vi "config-NTR.vi"() -> ()   [LabVIEW 2024]
uses:
  controls/UiNutritionPanel.ctl
  controls/UiScheduleTimestamp.ctl
  <vilib>/Utility/miscctls.llb/LVPointTypeDef.ctl
  controls/typePathSelector.ctl
  globals/globals-engine.vi
panel:
  in  "Index":u8=1 min=1 max=16 step=1
  in  "DataChanged?":bool=TRUE
  in  "Reload":bool
  in  "Save":bool
  in  "conf in":T1[](array[typedef]) {"ORP Dosing"."MIX Limit" format="%d [s]"; "ORP Dosing"."MIX Dose" format="%d [s]"; "PH Dosing"."ACID Limit" format="%d [s]"; "PH Dosing"."BASE Limit" format="%d [s]"; "PH Dosing"."ACID Dose" format="%d [s]"; "PH Dosing"."BASE Dose" format="%d [s]"; "EC Dosing"."BETA2 Limit" format="%d [s]"; "EC Dosing"."ALFA2 Limit" format="%d [s]"; "EC Dosing"."ALFA2 Dose" format="%d [s]"; "EC Dosing"."BETA2 Dose" format="%d [s]"; "EC Dosing"."BETA1 Limit" format="%d [s]"; "EC Dosing"."ALFA1 Limit" format="%d [s]"; "EC Dosing"."ALFA1 Dose" format="%d [s]"; "EC Dosing"."BETA1 Dose" format="%d [s]"; "Main"."DailyActivityHours"."Begin Time" format="ON:    %<%H:%M>T"; "Main"."DailyActivityHours"."End Time" format="OFF:    %<%H:%M>T"; "Main"."WashTimes"."Out" format="Wash out: %d [sec]"; "Main"."WashTimes"."In" format="Wash in: %d [sec]"; "Water Dosing"."Water Limit" format="%d [s]"; "Water Dosing"."Water Dose" format="%d [s]"}
  # "Water"
  # "EC"
  # "PH"
  # "ORP"
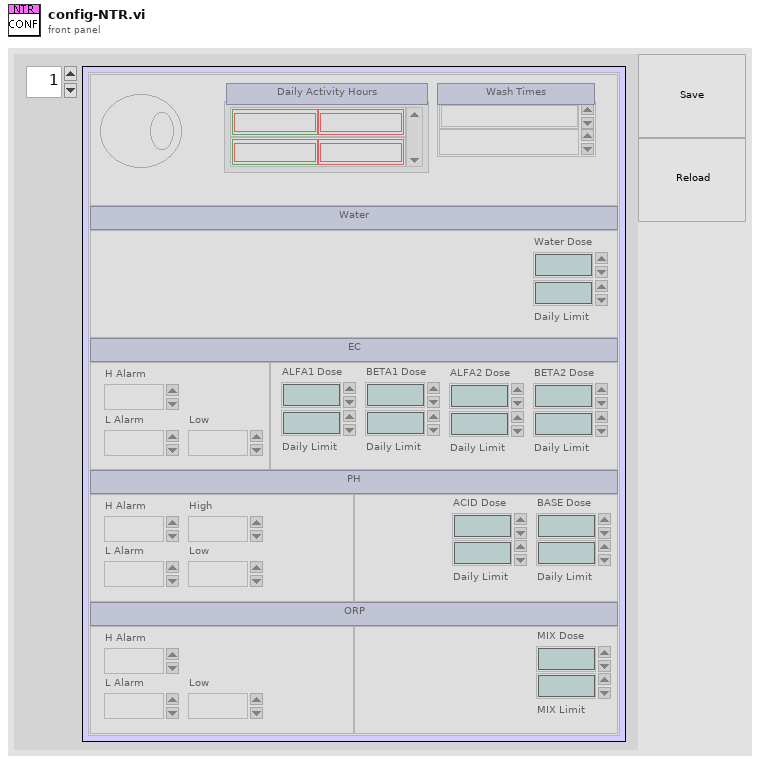
[diagram p1: front panel]
types:
  T1 = typedef "UiNutritionPanel.ctl" = cluster{"Main":cluster{"Enable":bool, "WashTimes":cluster{"In":dbl, "Out":dbl}, "DailyActivityHours":cluster{"Begin Time":T2, "End Time":T2}[]}, "Water Dosing":cluster{"Water Dose":dbl, "Water Limit":dbl}, "EC Ranges":cluster{"H Alarm":dbl, "L Alarm":dbl, "Low":dbl}, "EC Dosing":cluster{"ALFA1 Dose":dbl, "ALFA1 Limit":dbl, "BETA1 Dose":dbl, "BETA1 Limit":dbl, "ALFA2 Dose":dbl, "ALFA2 Limit":dbl, "BETA2 Dose":dbl, "BETA2 Limit":dbl}, "PH Ranges":cluster{"H Alarm":dbl, "L Alarm":dbl, "High":dbl, "Low":dbl}, "PH Dosing":cluster{"ACID Dose":dbl, "ACID Limit":dbl, "BASE Dose":dbl, "BASE Limit":dbl}, "ORP Ranges":cluster{"H Alarm":dbl, "L Alarm":dbl, "Low":dbl}, "ORP Dosing":cluster{"MIX Dose":dbl, "MIX Limit":dbl}}
  T2 = typedef "UiScheduleTimestamp.ctl" = timestamp
  T3 = typedef "typePathSelector.ctl" = enum16{"DIR_PROCS", "DIR_CONFIG", "DIR_TEMPLATE", "DIR_IO_FILE", "DIR_RECORD", "DIR_LOG", "DIR_RUNTIME", "DIR_PRESET", "DIR_INI"}
  T4 = typedef "LVPointTypeDef.ctl" = cluster{"Horizontal":i16, "Vertical":i16}
  T5 = enum32{"Invalid", "Standard", "Closed", "Hidden", "Minimized", "Maximized"}
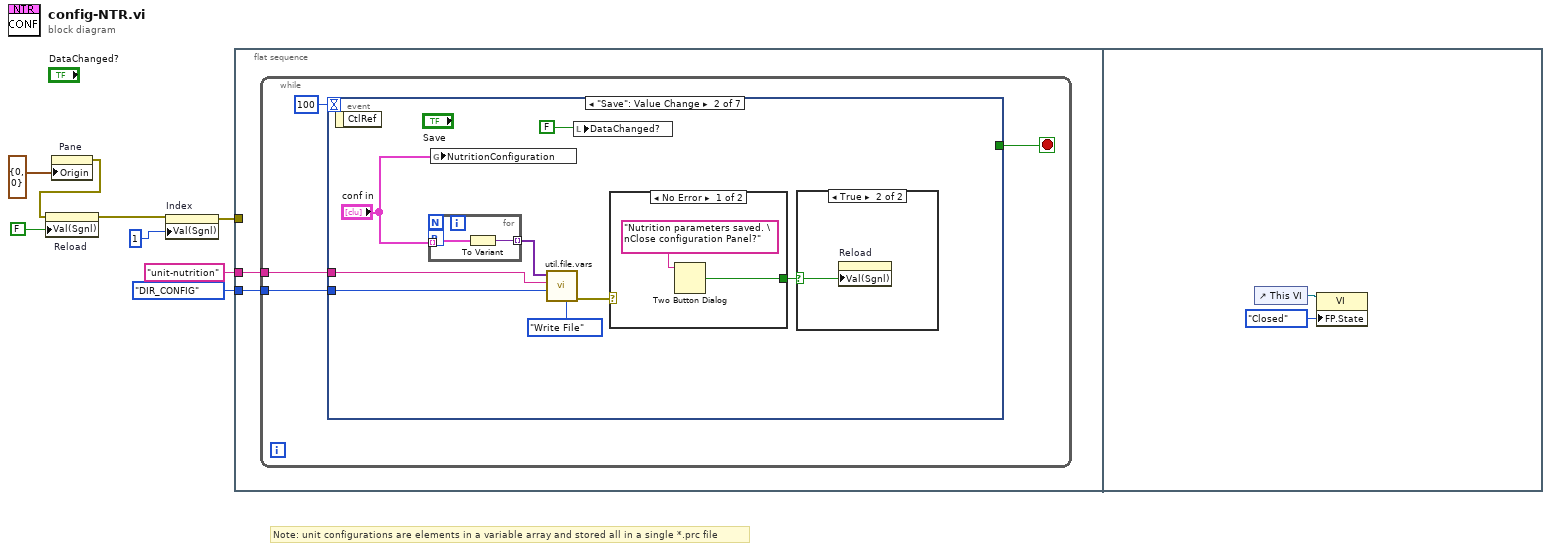
[diagram p0: block diagram]
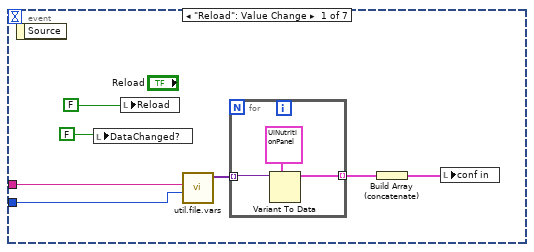
[diagram p2: hidden frame]
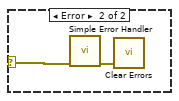
[diagram p4: hidden frame]
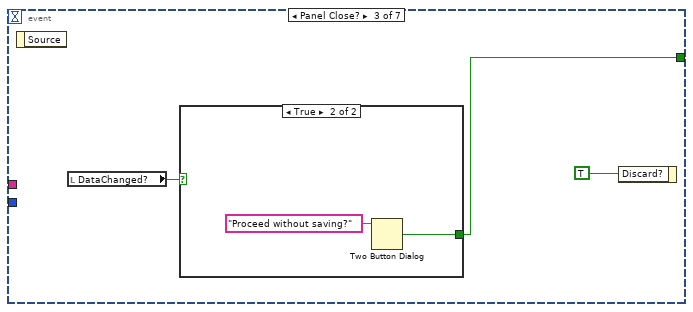
[diagram p5: hidden frame]
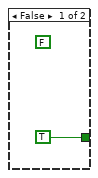
[diagram p6: hidden frame]
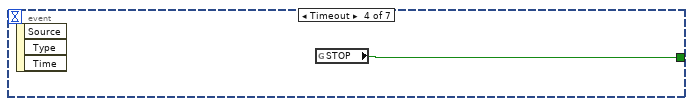
[diagram p7: hidden frame]
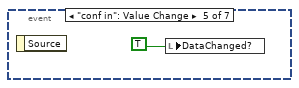
[diagram p8: hidden frame]
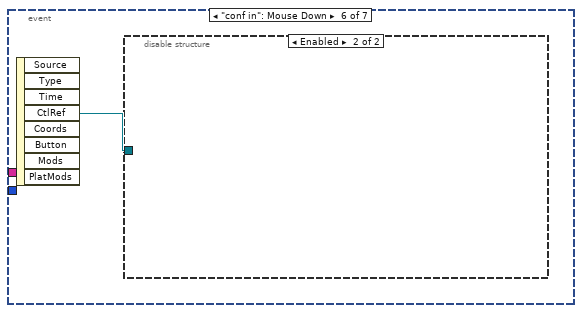
[diagram p9: hidden frame]
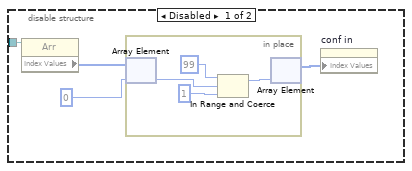
[diagram p10: hidden frame]
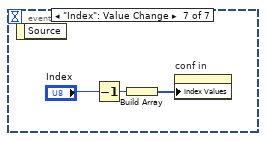
[diagram p11: hidden frame]
diagram:
  # "Note: unit configurations are elements in a variable array and stored all in a single *.prc file"
  n1 = property on="Pane" class="Pane"("Origin"=T4 {"Horizontal"=0, "Vertical"=0}) -> (error out=w1:errorcluster)  [unwired: 2 in, 1 out]
  n2 = property on="Reload" class="Bool (strict)"(error in=w1, "Val(Sgnl)"=FALSE ("Value (Signaling)")) -> (error out=w2:errorcluster)  [unwired: 1 in, 1 out]
  n3 = property on="Index" class="DigNum (strict)"(error in=w2, "Val(Sgnl)"=u8 1 ("Numeric")) -> (error out=w3:errorcluster)  [unwired: 1 in, 1 out]
  n4 = flat-sequence {
    tunnel: typePathSelector."DIR_CONFIG" ("location (PROCEDURE_DIR)") -> [w10]
    tunnel: "unit-nutrition" ("Filename.*  (opens dialog if empty and allow)") -> [w9]
    tunnel: w3 -> [_]
    frame #0 {
      n5 = while {
        tunnel: w10 -> [w14]
        tunnel: w9 -> [w13]
        stop <- w12 stop-if-true
        n6 = event shown="[1] \"Save\": Value Change" {
          selector: _ -> [_ _ _ _ _ _ _]
          dyn-events: _ -> [_ _ _ _ _ _ _]
          timeout: 100 -> [_ _ _ _ _ _ _]
          tunnel: w14 -> [w21 w31 _ _ _ _ _]
          tunnel: w13 -> [w20 w30 _ _ _ _ _]
          tunnel: [_ _ w41 w46 _ _ _] -> w12
          event "Reload": Value Change {
            n7 = event-data() -> ()  [unwired: 1 in, 1 out]
            n8 = local write "DataChanged?"(FALSE ("Value (Signaling)")) -> ()
            n9 = local write "Reload"(FALSE ("Reload")) -> ()
            n10 = call "util.file.vars.vi"("Directory (DIR_PROC)"=w21, "Proc Name(open dialog if empty)"=w20) -> ("Vars[] out"=w19:variant[])  [unwired: 5 in, 4 out]
            n11 = for {
              tunnel: w19 -> [w24] mode=indexing
              tunnel: [w23] -> w18 mode=indexing
              n12 = Variant To Data(type=T1 {"Main"={"Enable"=FALSE, "WashTimes"={"In"=0.0, "Out"=0.0}, "DailyActivityHours"=[]}, "Water Dosing"={"Water Dose"=0.0, "Water Limit"=0.0}, "EC Ranges"={"H Alarm"=0.0, "L Alarm"=0.0, "Low"=0.0}, "EC Dosing"={"ALFA1 Dose"=0.0, "ALFA1 Limit"=0.0, "BETA1 Dose"=0.0, "BETA1 Limit"=0.0, "ALFA2 Dose"=0.0, "ALFA2 Limit"=0.0, "BETA2 Dose"=0.0, "BETA2 Limit"=0.0}, "PH Ranges"={"H Alarm"=0.0, "L Alarm"=0.0, "High"=0.0, "Low"=0.0}, "PH Dosing"={"ACID Dose"=0.0, "ACID Limit"=0.0, "BASE Dose"=0.0, "BASE Limit"=0.0}, "ORP Ranges"={"H Alarm"=0.0, "L Alarm"=0.0, "Low"=0.0}, "ORP Dosing"={"MIX Dose"=0.0, "MIX Limit"=0.0}} ("Cluster"), Variant=w24) -> (data=w23:T1)  [unwired: 1 in, 1 out]
            }
            n13 = Build Array (concatenate)(w18) -> (w15:T1[])
            n14 = local write "conf in"(w15) -> ()
          }
          event "Save": Value Change {
            n15 = event-data() -> ()  [unwired: 1 in, 1 out]
            n16 = for {
              tunnel: "conf in" -> [w39] mode=indexing
              tunnel: [w38] -> w32 mode=indexing
              workers-P: _ -> [_]
              n17 = To Variant(anything=w39) -> (Variant=w38:variant)
            }
            n18 = global write "globals-engine.vi" "NutritionConfiguration"("conf in") -> ()
            n19 = call "util.file.vars.vi"("Operation(Read)"=enum16{"Read File", "Write File"}."Write File", "Directory (DIR_PROC)"=w31, "Proc Name(open dialog if empty)"=w30, "Vars[] in"=w32) -> ("error out"=w28:errorcluster)  [unwired: 3 in, 4 out]
            n20 = local write "DataChanged?"(FALSE ("Value (Signaling)")) -> ()
            n21 = case shown="No Error" w28 {
              selector: w28 -> [_ w37]
              tunnel: [w34 _] -> w27
              frame No Error {
                n22 = Two Button Dialog(message="Nutrition parameters saved. \nClose configuration Panel?") -> (T button?=w34:bool)  [unwired: 2 in]
              }
              frame Error {
                n23 = call <vilib>:"Simple Error Handler.vi"("error in (no error)"=w37) -> ("error out"=w36:errorcluster)  [unwired: 4 in, 4 out]
                n24 = call <vilib>:"Clear Errors.vi"("error in (no error)"=w36) -> ()  [unwired: 5 in, 2 out]
              }
            }
            n25 = case shown="True" w27 {
              selector: w27 -> [_ w33]
              frame False {
              }
              frame True {
                n26 = property on="Reload" class="Bool (strict)"("Val(Sgnl)"=w33) -> ()  [unwired: 2 in, 2 out]
              }
            }
          }
          event Panel Close? {
            n27 = event-data() -> ()  [unwired: 1 in, 1 out]
            n28 = local read "DataChanged?"() -> (w42:bool)
            n29 = case shown="True" w42 {
              tunnel: [TRUE ("T button?") w44] -> w41
              frame False {
                (unwired) FALSE ("T button?")
              }
              frame True {
                n30 = Two Button Dialog(message="Proceed without saving?") -> (T button?=w44:bool)  [unwired: 2 in]
              }
            }
            n31 = event-data("Discard?"=TRUE) -> ()  [unwired: 1 in, 1 out]
          }
          event Timeout {
            n32 = event-data() -> ()  [unwired: 1 in, 3 out]
            n33 = global read "globals-engine.vi" "STOP"() -> (w46:bool)
          }
          event "conf in": Value Change {
            n34 = event-data() -> ()  [unwired: 1 in, 1 out]
            n35 = local write "DataChanged?"(TRUE ("Value (Signaling)")) -> ()
          }
          event "conf in": Mouse Down {
            n36 = event-data() -> ("CtlRef"=w48:refnum<vi>)  [unwired: 1 in, 7 out]
            n37 = disable-structure shown="Enabled" {
              disable-tunnel: w48 -> [w50 _]
              frame Disabled {
                n38 = property class="Arr"(reference=w50) -> ("Index Values"=w49:u32[])  [unwired: 1 in, 2 out]
                n39 = in-place {
                  n40 = in-place-array #1(w49, 0) -> (w56:u32)
                  n41 = In Range and Coerce(upper limit=99, x=w56, lower limit=u32 1) -> (coerced(x)=w54:u32)  [unwired: 1 out]
                  n42 = in-place-array #1(w54) -> (w51:u32[])  [unwired: 1 out]
                }
                n43 = property on="conf in" class="Arr"("Index Values"=w51) -> ()  [unwired: 2 in, 2 out]
              }
              frame Enabled {
              }
            }
          }
          event "Index": Value Change {
            n44 = event-data() -> ()  [unwired: 1 in, 1 out]
            n45 = Decrement(x="Index") -> (x-1=w57:u8)
            n46 = Build Array(w57) -> (w58:u8[])
            n47 = property on="conf in" class="Arr"("Index Values"=w58) -> ()  [unwired: 2 in, 2 out]
          }
        }
      }
    }
    frame #1 {
      n48 = control-ref of="This VI"() -> (w61:refnum<vi>)
      n49 = property class="VI"(reference=w61, "FP.State"=T5."Closed" ("Front Panel Window:State")) -> ()  [unwired: 1 in, 2 out]
    }
  }
